vi "Division of Polynomials (CDB).vi"(9 "q":cdb[](array[numeric]), 11 "p":cdb[](array[numeric])) -> (1 "rest":cdb[](array[numeric]), 3 "p/q":cdb[](array[numeric]))   [LabVIEW 2018, in "NI_AALPro.lvlib"]
uses:
  NI_AALPro.lvlib
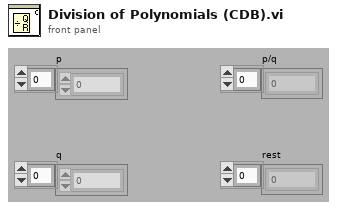
[diagram p1: front panel]
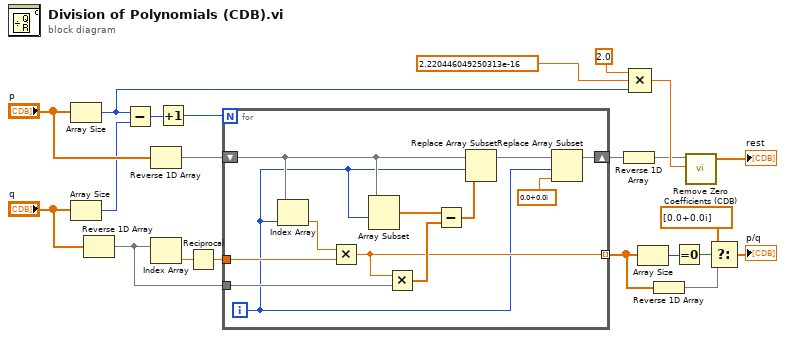
[diagram p0: block diagram]
diagram:
  n1 = Array Size(array="p") -> (size(s)=w12:i32)
  n2 = Array Size(array="q") -> (size(s)=w18:i32)
  n3 = Reverse 1D Array(array="q") -> (reversed array=w5:cdb[])
  n4 = Subtract(x=w12, y=w18) -> (x-y=w22:i32)
  n5 = Reverse 1D Array(array="p") -> (reversed array=w7:cdb[])
  n6 = Index Array(array=w5) -> (element=w1:cdb)  [unwired: 1 in]
  n7 = Increment(x=w22) -> (x+1=w21:i32)
  n8 = Reciprocal(x=w1) -> (1/x=w2:cdb)
  n9 = for {
    N: w21 -> [_]
    shift-right: [w27] -> w4
    shift-left: w7 -> [w31]
    tunnel: w5 -> [w24]
    tunnel: w2 -> [w33]
    tunnel: [w25] -> w6 mode=indexing
    i -> [w23]
    n10 = Index Array(array=w31, index=w23) -> (element=w34:cdb)
    n11 = Multiply(x=w34, y=w33) -> (x*y=w25:cdb)
    n12 = Array Subset(array=w31, index=w23) -> (w26:cdb[])  [unwired: 1 in]
    n13 = Multiply(x=w25, y=w24) -> (x*y=w32:cdb[])
    n14 = Subtract(x=w26, y=w32) -> (x-y=w30:cdb[])
    n15 = Replace Array Subset(array=w31, new element=w30, index=w23) -> (w29:cdb[])
    n16 = Replace Array Subset(array=w29, new element=cdb 0.0+0.0i ("new element/subarray"), index=w23) -> (w27:cdb[])
  }
  n17 = Reverse 1D Array(array=w4) -> (reversed array=w3:cdb[])
  n18 = Compound Arithmetic op=MULTIPLY(2.0, 2.220446049250313e-16 ("eps for remove zeros"), w12) -> (w9:dbl)
  n19 = Array Size(array=w6) -> (size(s)=w17:i32)
  n20 = Reverse 1D Array(array=w6) -> (reversed array=w14:cdb[])
  n21 = Equal To 0?(x=w17) -> (x = 0?=w16:bool)
  n22 = call "Remove Zero Coefficients (CDB).vi"("threshold"=w9, "P(x) In"=w3) -> ("P(x) Out"=→"rest":cdb[])  [unwired: 7 in, 2 out]
  n23 = Select(t=cdb[] [0.0+0.0i], s=w16, f=w14) -> (s? t:f=→"p/q":cdb[])
